vi "Map to Tree.vi"(10 "Tree":refnum<vi>, 11 "Map in":map{string[], T1}(c390)) -> ()   [LabVIEW 2020, in "VolatusDAQGenericGUI.lvlib" / "GenericGuiAI.lvclass"]
uses:
  GenericGuiAI.lvclass
  AI Tree Entry.ctl
  Channel Entry.ctl
  GenericGuiAI.lvclass/GenericGuiAI.ctl
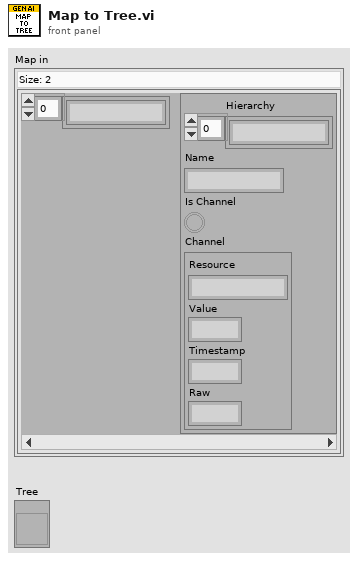
[diagram p1: front panel]
types:
  T1 = typedef "VolatusDAQGenericGUI.lvlib/GenericGuiAI.lvclass/AI Tree Entry.ctl" = cluster{"Hierarchy":string[], "Name":string, "Is Channel":bool, "Channel":T2}
  T2 = typedef "VolatusDAQGenericGUI.lvlib/GenericGuiAI.lvclass/Channel Entry.ctl" = cluster{"Resource":string, "Value":dbl, "Timestamp":dbl, "Raw":dbl}
  T3 = typedef "LVNodeAndColumnTypeDef.ctl" = cluster{"Node":string, "Column":i32}
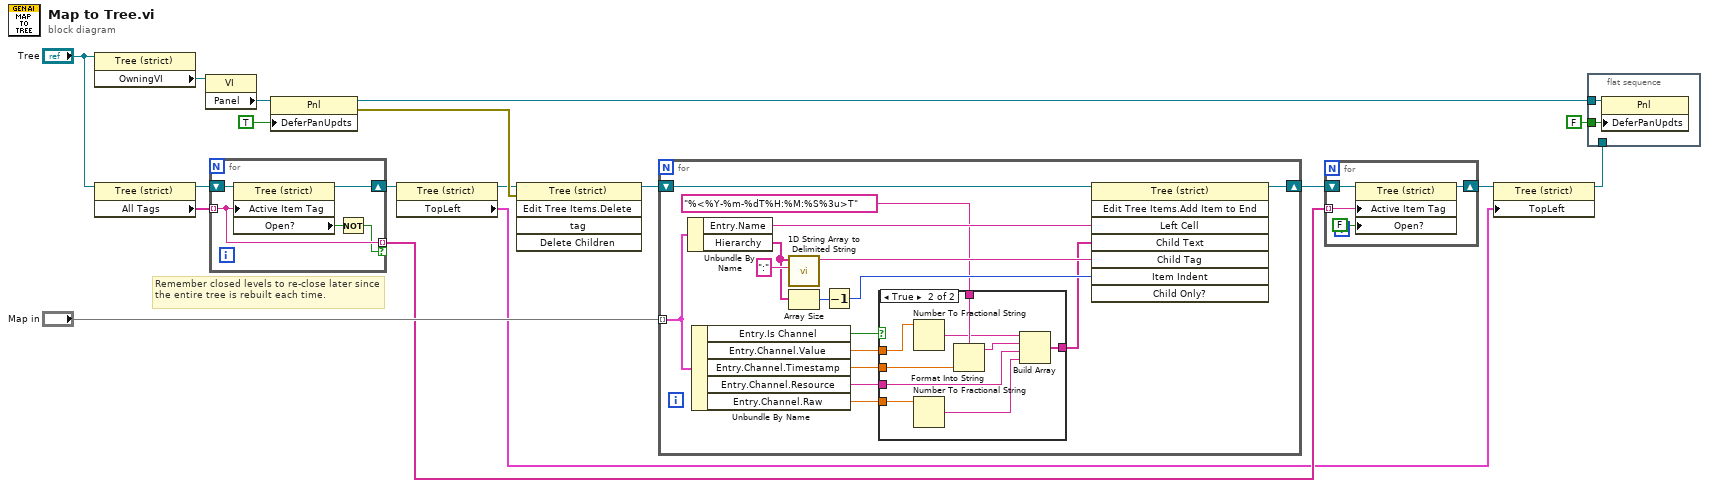
[diagram p0: block diagram]
diagram:
  # "Remember closed levels to re-close later since the entire tree is rebuilt each time."
  n1 = property class="Tree (strict)"(reference="Tree") -> ("OwningVI"=w17:refnum<vi>)  [unwired: 1 in, 2 out]
  n2 = property class="Tree (strict)"(reference="Tree") -> (reference out=w13:refnum<vi>, "All Tags"=w12:string[])  [unwired: 1 in, 1 out]
  n3 = property class="VI"(reference=w17) -> ("Panel"=w16:refnum<vi>)  [unwired: 1 in, 2 out]
  n4 = for {
    shift-right: [w19] -> w11
    shift-left: w13 -> [w23]
    tunnel: w12 -> [w21] mode=indexing
    tunnel: [w21] -> w5 mode=indexing if=w20
    n5 = property class="Tree (strict)"(reference=w23, "Active Item Tag"=w21) -> (reference out=w19:refnum<vi>, "Open?"=w22:bool)  [unwired: 1 in, 1 out]
    n6 = Not(x=w22) -> (.not. x?=w20:bool)
  }
  n7 = property class="Pnl"(reference=w16, "DeferPanUpdts"=TRUE ("Defer Panel Updates")) -> (reference out=w2:refnum<vi>, error out=w18:errorcluster)  [unwired: 1 in]
  n8 = property class="Tree (strict)"(reference=w11) -> (reference out=w10:refnum<vi>, "TopLeft"=w4:T3)  [unwired: 1 in, 1 out]
  n9 = invoke class="Tree (strict)" method="Edit Tree Items.Delete"(reference=w10, error in=w18) -> (reference out=w9:refnum<vi>)  [unwired: 3 in, 4 out]
  n10 = for {
    shift-right: [w31] -> w6
    shift-left: w9 -> [w39]
    tunnel: "Map in" -> [w32] mode=indexing
    n11 = Unbundle By Name(w32) -> ("Entry.Name"=w38:string, "Hierarchy"=w35:string[])
    n12 = Unbundle By Name(w32) -> ("Entry.Is Channel"=w24:bool, "Entry.Channel.Value"=w30:dbl, "Entry.Channel.Timestamp"=w28:dbl, "Entry.Channel.Resource"=w27:string, "Entry.Channel.Raw"=w26:dbl)
    n13 = call <vilib>:"1D String Array to Delimited String.vi"("delimiter"=":", "string array"=w35) -> ("delimited string"=w36:string)  [unwired: 9 in]
    n14 = Array Size(array=w35) -> (size(s)=w34:i32)
    n15 = Decrement(x=w34) -> (x-1=w33:i32)
    n16 = case shown="True" w24 {
      tunnel: w30 -> [_ w48]
      tunnel: "%<%Y-%m-%dT%H:%M:%S%3u>T" -> [_ w47]
      tunnel: w28 -> [_ w46]
      tunnel: w27 -> [_ w43]
      tunnel: w26 -> [_ w42]
      tunnel: [_ w40] -> w25
      frame False {
      }
      frame True {
        n17 = Number To Fractional String(number=w48) -> (F-format string=w45:string)  [unwired: 3 in]
        n18 = Number To Fractional String(number=w42) -> (F-format string=w41:string)  [unwired: 3 in]
        n19 = Format Into String(format string=w47, w46) -> (resulting string=w44:string)  [unwired: 2 in, 1 out]
        n20 = Build Array(w45, w44, w43, w41) -> (w40:string[])
      }
    }
    n21 = invoke class="Tree (strict)" method="Edit Tree Items.Add Item to End"(reference=w39, "Left Cell"=w38, "Child Text"=w25, "Child Tag"=w36, "Item Indent"=w33) -> (reference out=w31:refnum<vi>)  [unwired: 3 in, 7 out]
  }
  n22 = for {
    shift-right: [w51] -> w7
    shift-left: w6 -> [w52]
    tunnel: w5 -> [w49] mode=indexing
    n23 = property class="Tree (strict)"(reference=w52, "Active Item Tag"=w49, "Open?"=FALSE ("Active Item:Open?")) -> (reference out=w51:refnum<vi>)  [unwired: 1 in, 1 out]
  }
  n24 = property class="Tree (strict)"(reference=w7, "TopLeft"=w4) -> (reference out=w1:refnum<vi>)  [unwired: 1 in, 1 out]
  n25 = flat-sequence {
    tunnel: FALSE ("Defer Panel Updates") -> [w54]
    tunnel: w2 -> [w53]
    tunnel: w1 -> [_]
    frame #0 {
      n26 = property class="Pnl"(reference=w53, "DeferPanUpdts"=w54) -> ()  [unwired: 1 in, 2 out]
    }
  }
